vi "WB_NextStep.vi"(8 "error in (no error)":errorcluster, 10 "Properties":T2, 11 "Previous Step":T1) -> (0 "error out":errorcluster, 3 "Next Step":T1)   [LabVIEW 2019]
uses:
  Communication/TypeDef/#TypeDef_FromMRtoPC.ctl
  Communication/TypeDef/#TypeDef_FromPCtoMR.ctl
  Communication/TypeDef/#TypeDef_Command.ctl
  Communication/TypeDef/#TypeDef_ErrorHandler_prop.ctl
  TypeDef/#TypeDef_EnumOp_WebServer.ctl
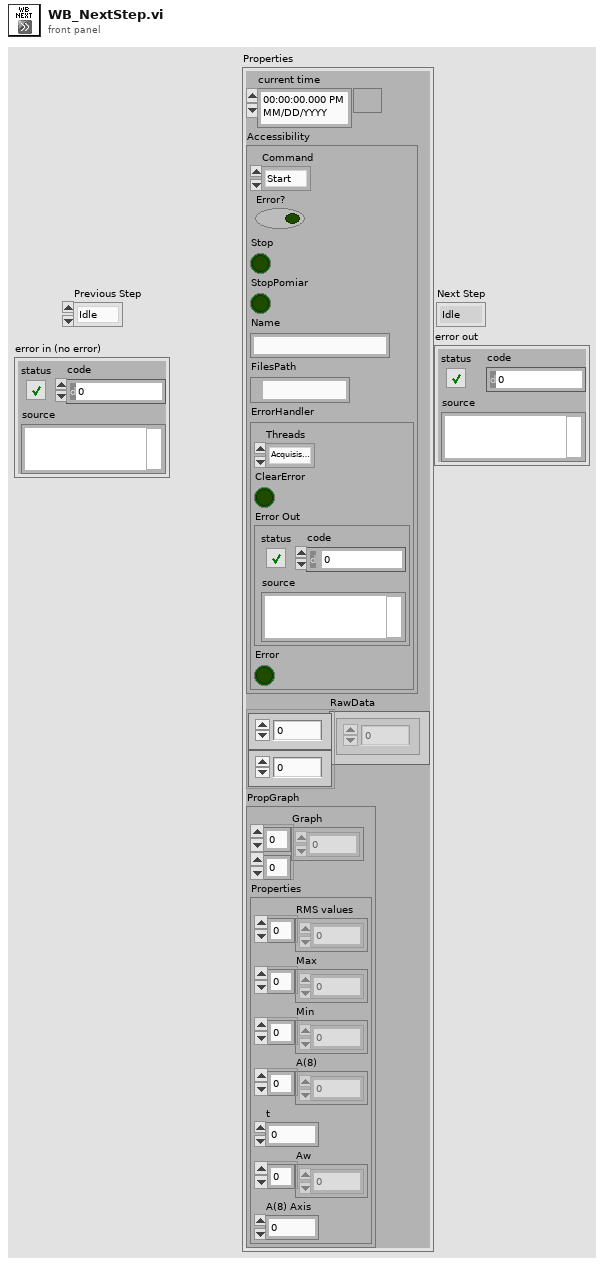
[diagram p1: front panel]
types:
  T1 = typedef "#TypeDef_EnumOp_WebServer.ctl" = enum16{"Idle", "Init", "Sharing", "End", "Error_Shutdown", "ClearError"}
  T2 = typedef "#TypeDef_FromMRtoPC.ctl" = cluster{"current time":timestamp, "Accessibility":T3, "RawData":dbl[][], "PropGraph":cluster{"Graph":dbl[][], "Properties":cluster{"RMS values":dbl[], "Max":dbl[], "Min":dbl[], "A(8)":dbl[], "t":dbl, "Aw":dbl[], "A(8) Axis":dbl}}}
  T3 = typedef "#TypeDef_FromPCtoMR.ctl" = cluster{"Command":T4, "Error?":bool, "Stop":bool, "StopPomiar":bool, "Name":string, "FilesPath":path, "ErrorHandler":T5}
  T4 = typedef "#TypeDef_Command.ctl" = enum16{"Start", "End"}
  T5 = typedef "#TypeDef_ErrorHandler_prop.ctl" = cluster{"Threads":enum16{"Acquisistion", "Data Operation", "Save File"}, "ClearError":bool, "Error Out ":errorcluster, "Error":bool}
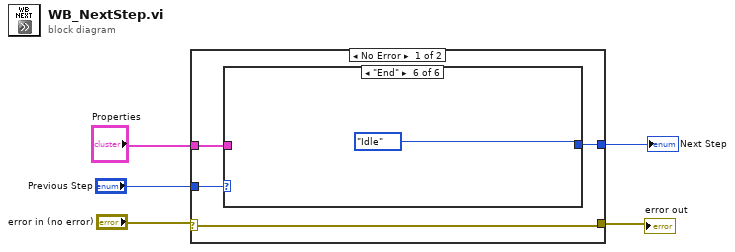
[diagram p0: block diagram]
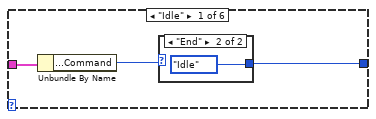
[diagram p2: hidden frame]
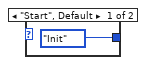
[diagram p3: hidden frame]
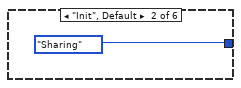
[diagram p4: hidden frame]
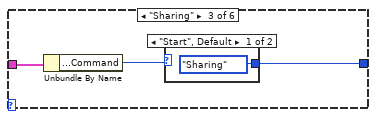
[diagram p5: hidden frame]
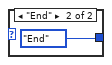
[diagram p6: hidden frame]
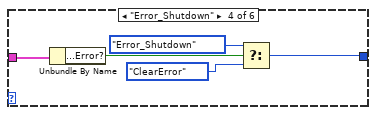
[diagram p7: hidden frame]
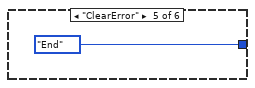
[diagram p8: hidden frame]
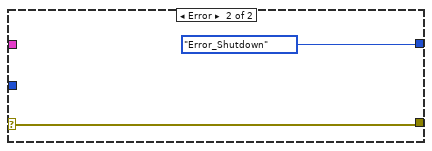
[diagram p9: hidden frame]
diagram:
  n1 = case shown="No Error" "error in (no error)" {
    selector: "error in (no error)" -> [w6 w29]
    tunnel: [w6 w29] -> w4
    tunnel: [w9 #TypeDef_EnumOp_WebServer."Error_Shutdown" ("EnumOp_DataAcquisition")] -> w1
    tunnel: "Properties" -> [w8 _]
    tunnel: "Previous Step" -> [w7 _]
    frame No Error {
      n2 = case shown="\"End\"" w7 {
        tunnel: w8 -> [w11 _ w17 w25 _ _]
        tunnel: [w10 #TypeDef_EnumOp_WebServer."Sharing" ("EnumOp_DataAcquisition") w16 w24 #TypeDef_EnumOp_WebServer."End" ("EnumOp_DataAcquisition") #TypeDef_EnumOp_WebServer."Idle" ("EnumOp_DataAcquisition")] -> w9
        frame "Idle" {
          n3 = Unbundle By Name(w11) -> ("Accessibility.Command"=w12:T4)
          n4 = case shown="\"End\"" w12 {
            tunnel: [#TypeDef_EnumOp_WebServer."Init" ("EnumOp_DataAcquisition") #TypeDef_EnumOp_WebServer."Idle" ("EnumOp_DataAcquisition")] -> w10
            frame "Start", Default {
            }
            frame "End" {
            }
          }
        }
        frame "Init", Default {
        }
        frame "Sharing" {
          n5 = Unbundle By Name(w17) -> ("Accessibility.Command"=w18:T4)
          n6 = case shown="\"Start\", Default" w18 {
            tunnel: [#TypeDef_EnumOp_WebServer."Sharing" ("EnumOp_DataAcquisition") #TypeDef_EnumOp_WebServer."End" ("EnumOp_DataAcquisition")] -> w16
            frame "Start", Default {
            }
            frame "End" {
            }
          }
        }
        frame "Error_Shutdown" {
          n7 = Unbundle By Name(w25) -> ("Accessibility.Error?"=w23:bool)
          n8 = Select(t=#TypeDef_EnumOp_WebServer."Error_Shutdown" ("EnumOp_DataAcquisition"), s=w23, f=#TypeDef_EnumOp_WebServer."ClearError" ("EnumOp_DataAcquisition")) -> (s? t:f=w24:T1)
        }
        frame "ClearError" {
        }
        frame "End" {
        }
      }
    }
    frame Error {
    }
  }
  "error out" <- w4
  "Next Step" <- w1
